vi "STEP LOAD SEQUENCE.vi"(8 "error in (no error)":errorcluster, 11 "main ref":T1) -> (0 "error out":errorcluster)   [LabVIEW 2025]
uses:
  controls/LAB-IQ UI Data.ctl
  STEP LOAD SEQUENCE ENUM.ctl
  HEAVE vi's/Heave Write enum.ctl
  cef93557-1e48-4b46-994d-460df1ebe7ff.vi
panel:
  out "ELAPSED TIMER":dbl
  out "Test Size":i32
  in  "Time Index":i32
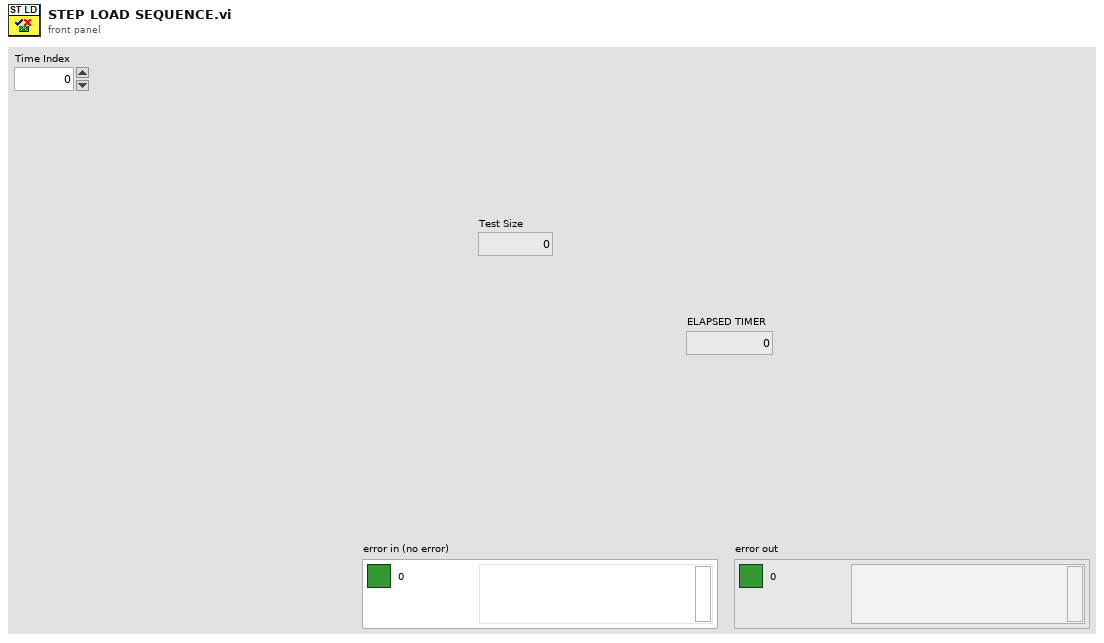
[diagram p1: front panel]
types:
  T1 = typedef "LAB-IQ UI Data.ctl" = cluster{"Main Home Screen":cluster{"GUI":refnum<vi>, "Platform Settings":refnum<vi>, "Configure":refnum<vi>, "Home":refnum<vi>, "EXIT":refnum<vi>, "service 2":refnum<vi>, "MainPage":refnum<vi>, "Analysis":refnum<vi>}, "Platform Settings":cluster{"mm/s  Surge":refnum<vi>, "Update Surge Speed":refnum<vi>, "Drive Error":refnum<vi>, "Disable Axis Jog Soft Limits":refnum<vi>, "mm/s  Sway":refnum<vi>, "Sway and Surge COM Status":refnum<vi>, "Heave COM Status":refnum<vi>, "Enable Platform":refnum<vi>, "Surge Forward Main":refnum<vi>, "Sway Right Main":refnum<vi>, "Sway Left Main":refnum<vi>, "Heave Down Main":refnum<vi>, "Heave Up main":refnum<vi>, "Update Sway Speed":refnum<vi>, "Update Heave Speed":refnum<vi>, "mm/s Heave":refnum<vi>, "mm/sec":refnum<vi>, "mm":refnum<vi>, "Surge Backward Main":refnum<vi>}, "Analysis Screen":cluster{"Analysis Home":refnum<vi>, "Surface Analysis":refnum<vi>, "Imaging":refnum<vi>, "Image Analysis":refnum<vi>, "Post Analysis":refnum<vi>}, "Config Screen":cluster{"Select Load Head":refnum<vi>, "Notes :":refnum<vi>, "FILE":refnum<vi>, "Sample ID :":refnum<vi>, "Operator ID :":refnum<vi>, "Operator Name :":refnum<vi>, "Auto":refnum<vi>}, "Motion Module":cluster{"zNL":refnum<vi>, "NL disp":refnum<vi>, "Rotary Tab":refnum<vi>, "Motion Direction:  3":refnum<vi>, "E.Velocity 2":refnum<vi>, "e.v/ssr 2":refnum<vi>, "Enter Fixed E.Velocity 2":refnum<vi>, "Enter Final SRR 2":refnum<vi>, "Enter initial SRR 2":refnum<vi>, "Enter Fixed SRR 2":refnum<vi>, "Enter the Final E.Velocity (m/s) 2":refnum<vi>, "Enter initial E.Velocity (m/s) 2":refnum<vi>, "Final Speed (RPM) 3":refnum<vi>, "Initial Speed (RPM) 2":refnum<vi>, "Enter the Final Velocity (m/s) 3":refnum<vi>, "Enter initial Velocity (m/s)  3":refnum<vi>, "Ramp Up 2":refnum<vi>, "TEST SELECTION":refnum<vi>, "SPEED SELECTION : ":refnum<vi>, "Angular Oscillation Set":refnum<vi>, "Traction":refnum<vi>, "Step Speed":refnum<vi>, "StepTable For Load-Speed":refnum<vi>, "StepTable For Speed":refnum<vi>, "Surge Forward MM":refnum<vi>, "Surge Backward MM":refnum<vi>, "M3 Image":refnum<vi>, "String 39":refnum<vi>, "Sway Left MM":refnum<vi>, "Sway Right MM":refnum<vi>, "Disable Axis Jog Soft Limits":refnum<vi>, "mm":refnum<vi>, "Heave Down MM":refnum<vi>, "Heave Up MM":refnum<vi>, "Wear Track Diameter (mm)":refnum<vi>, "Set WTD":refnum<vi>, "HomeScratch":refnum<vi>, "HomeRot":refnum<vi>, "PlaceModule":refnum<vi>, "Enter the Angle (Deg)":refnum<vi>, "Enter the Frequency (Hz)":refnum<vi>, "Motion Mode:":refnum<vi>, "LR Sway":refnum<vi>, "Rot Hor":refnum<vi>, "Scratch":refnum<vi>, "LR Cam":refnum<vi>, "MMBack":refnum<vi>, "MMNext":refnum<vi>, "Rot Ver":refnum<vi>, "Rotary Module Selection":refnum<vi>, "calculate rotary":refnum<vi>, "SPEED SELECTION : rotary":refnum<vi>, "Import 2":refnum<vi>, "Save 2":refnum<vi>, "File Path :  2":refnum<vi>, "String 45":refnum<vi>, "StepTable For Speed 3":refnum<vi>, "Enter the Speed(mm/sec)":refnum<vi>, "Enter the Speed(RPM)":refnum<vi>, "Enter Scratch Speed (mm/s):":refnum<vi>, "SwaySpeed Set":refnum<vi>, "Scartch Offset":refnum<vi>, "Motion type:":refnum<vi>, "HomeScratch 2":refnum<vi>, "Enter Scratch length (mm):":refnum<vi>, "Wear Track Diameter":refnum<vi>, "Rotary Speed Exced":refnum<vi>, "Scratch Mode":refnum<vi>, "No of Scratch":refnum<vi>}, "Environmental control":cluster{"Humidity  Status  3":refnum<vi>, "Low Temp  Status  2":refnum<vi>, "TK4 status 2":refnum<vi>, "Stage Temperature":refnum<vi>, "Sample Temperature":refnum<vi>, "Humidity (Amb)":refnum<vi>, "Clear List":refnum<vi>, "Add to list":refnum<vi>, "Wear":refnum<vi>, "Vibration":refnum<vi>, "Humidity (Chamber)":refnum<vi>, "Temperature (Chamber)":refnum<vi>, "ECR ":refnum<vi>, "Temperature (Amb)":refnum<vi>, "Microphone":refnum<vi>, "Acoustic Emission 3":refnum<vi>, "SNext":refnum<vi>, "APBack":refnum<vi>, "Enter the Temperature (°C):":refnum<vi>, "Enter the Stage \nTemperature (°C):":refnum<vi>, "Enter the Humidity (%Rh):":refnum<vi>, "Low Temp":refnum<vi>, "High Temp":refnum<vi>, "Humidity":refnum<vi>, "Sensors Picked":refnum<vi>}, "About Screen":cluster{"Password":refnum<vi>, "Home Service":refnum<vi>, "Advanced Setting":refnum<vi>, "About Tab":refnum<vi>, "ECR Port:":refnum<vi>, "Ramp Port:":refnum<vi>, "Installation/Replacement completed":refnum<vi>, "Loahead":refnum<vi>, "Heave and Surge COM Port:":refnum<vi>, "Sway COM Port:":refnum<vi>, "Temp Modbus:":refnum<vi>, "Humidity Port:":refnum<vi>, "Edit Gain Constants":refnum<vi>, "Save Gain Constants":refnum<vi>}, "Main Screen":cluster{"Main Screen Tab":refnum<vi>, "Angle and Frequency":refnum<vi>, "Stroke (mm)":refnum<vi>, "Angle (Deg)":refnum<vi>, "Main Speed Tab":refnum<vi>, "MTM MOTOR DISPLAY":refnum<vi>, "Disc Speed (m/sec)":refnum<vi>, "Ball Speed (m/sec)":refnum<vi>, "Disc Speed (RPM)":refnum<vi>, "Ball Speed (RPM)":refnum<vi>, "SPEED TAB":refnum<vi>, "Speed (m/sec)":refnum<vi>, "Set Speed (m/sec)":refnum<vi>, "Speed (RPM)":refnum<vi>, "Set Speed":refnum<vi>, "Time Tab":refnum<vi>, "Time ( HH:MM:SS ) 2":refnum<vi>, "Test Duration":refnum<vi>, "Test Duration 4":refnum<vi>, "TEST CYCLE":refnum<vi>, "TOTAL CYCLES":refnum<vi>, "Set Load (N)":refnum<vi>, "Temp Tabs":refnum<vi>, "Heater":refnum<vi>, "TK4 status":refnum<vi>, "ChamberTemp":refnum<vi>, "SetTmp":refnum<vi>, "Controller  Status":refnum<vi>, "ChamberTemp 2":refnum<vi>, "SetTmp 2":refnum<vi>, "Controller  Status 2":refnum<vi>, "ChamberTemp 3":refnum<vi>, "SetTmp 3":refnum<vi>, "Cooling":refnum<vi>, "Load Communication":refnum<vi>, "Ambient \nTemperature":refnum<vi>, "HumCOMStatus":refnum<vi>, "Ambient\n Humidity":refnum<vi>, "Freq (Hz)":refnum<vi>, "Load En":refnum<vi>, "NLt":refnum<vi>, "zNL 2":refnum<vi>, "Humidity On":refnum<vi>, "humidity disp":refnum<vi>, "Set Humidity":refnum<vi>, "NL disp 2":refnum<vi>, "Humidity On 2":refnum<vi>, "humidity disp 2":refnum<vi>, "Set Humidity 2":refnum<vi>, "NL disp 3":refnum<vi>, "AppLoadSeq scratch":refnum<vi>, "Stop Scratch":refnum<vi>, "ClrLog":refnum<vi>, "Trip Log":refnum<vi>, "STOP":refnum<vi>, "Start Test":refnum<vi>, "Test status":refnum<vi>, "AR Led":refnum<vi>, "Data":refnum<vi>, "Health":refnum<vi>, "Sway COM Status":refnum<vi>, "Heave COM Status":refnum<vi>, "Grp Tab":refnum<vi>, "Sub Graph":refnum<vi>, "SD (mm)":refnum<vi>, "Siliding distance Reset Graph":refnum<vi>, "SDGp":refnum<vi>, "Humidity Reset Graph":refnum<vi>, "HumrGp":refnum<vi>, "Acoustic Emission (mV)":refnum<vi>, "Aqucostic Reset Graph":refnum<vi>, "gACQUOS":refnum<vi>, "ECR RESET":refnum<vi>, "ECR":refnum<vi>, "Temperature Reset":refnum<vi>, "Acoustic Emission (mV) 2":refnum<vi>, "Aqucostic Reset Graph 2":refnum<vi>, "gACQUOS 2":refnum<vi>, "ECR RESET 2":refnum<vi>, "ECR 2":refnum<vi>, "Temperature Reset 2":refnum<vi>, "Temperature (deg c)":refnum<vi>, "Speed Reset Graph":refnum<vi>, "Speed Tab":refnum<vi>, "MTM DISC  SPEED":refnum<vi>, "MTM BALL SPEED":refnum<vi>, "speed mm/sec":refnum<vi>, "Hymidity":refnum<vi>, "Humidity Disable trip":refnum<vi>, "CoF Trip  2":refnum<vi>, "Depth Trip":refnum<vi>, "Weart Deapth":refnum<vi>, "Depth Reset Graph":refnum<vi>, "Weart":refnum<vi>, "Depthz":refnum<vi>, "Depth (µm)":refnum<vi>, "WearGp":refnum<vi>, "NL Trip 2":refnum<vi>, "Load pid":refnum<vi>, "Load Disable Trip":refnum<vi>, "Load Reset Graph":refnum<vi>, "NL Display 4":refnum<vi>, "Main Chart 3":refnum<vi>, "BACK":refnum<vi>, "Depth Trip 2":refnum<vi>, "COF TRIP ":refnum<vi>, "Friction Force (N)":refnum<vi>, "FF Reset Graph":refnum<vi>, "FF Disable Trip":refnum<vi>, "FF TRIP":refnum<vi>, "COF Disable Trip":refnum<vi>, "COF Reset Graph":refnum<vi>, "Start Test Temp":refnum<vi>, "zFF":refnum<vi>, "Friction Force (N) Graph":refnum<vi>, "Coefficient of Friction":refnum<vi>, "Scratch Start Test":refnum<vi>, "FF Tab":refnum<vi>, "Cyclic Friction Force (N)":refnum<vi>, "CZ FF":refnum<vi>, "Cyclic Friction Force (N) Graph":refnum<vi>, "Cyclic Coefficient of Friction":refnum<vi>, "Cyclic FF TRIP":refnum<vi>, "Cyclic FF Disable Trip":refnum<vi>, "cyclic COF Disable Trip":refnum<vi>, "cyclic COF TRIP":refnum<vi>, "cyclic COF Reset Graph":refnum<vi>, "Cyclic FF Reset Graph":refnum<vi>, "Test Trip":refnum<vi>, "Multi Scratch Pass":refnum<vi>}, "Loading":cluster{"Indentation":refnum<vi>, "Reference Sample":refnum<vi>, "Load Cell Communication Slide":refnum<vi>, "com 3":refnum<vi>, "com":refnum<vi>, "DecaForce COM Status":refnum<vi>, "Update":refnum<vi>, "Clear 3":refnum<vi>, "seq":refnum<vi>, "Stribeck table":refnum<vi>, "Stribeck Table  For loading":refnum<vi>, "Loading Mode":refnum<vi>, "Enter the Final Load (N)":refnum<vi>, "Enter the CoF Trip":refnum<vi>, "Enter the Friction Force Trip":refnum<vi>, "Enter the Normal load Trip":refnum<vi>, "Enter the Load  (N)":refnum<vi>, "KiloForce":refnum<vi>, "DecaForce ":refnum<vi>, "MicroForce":refnum<vi>, "LHBack":refnum<vi>, "LHNext":refnum<vi>, "Enter the Loading Rate (N/min)":refnum<vi>, "Message":refnum<vi>, "Warning 2":refnum<vi>, "SSP 0.75":refnum<vi>, "SSP 0.5":refnum<vi>, "SSP 0.3":refnum<vi>, "Warning":refnum<vi>, "gui GIF":refnum<vi>, "Communication is established":refnum<vi>, "AppLoad 4":refnum<vi>, "Multipoint":refnum<vi>, "Load Selection":refnum<vi>}, "PID":cluster{"Ramp MulFac":refnum<vi>, "pulses LoadDiffRamp(2..10)":refnum<vi>, "PulseControlRamp(diff<=3N)":refnum<vi>, "SetLoadDeadband(%) Load(0-10N)":refnum<vi>, "PID gains out delay (microForce)":refnum<vi>, "Ramp":refnum<vi>, "Gain 2":refnum<vi>, "pulses LoadDiff(2..10)":refnum<vi>, "pulses LoadDiff(11..50)":refnum<vi>, "PulseControl(diff<=3N)":refnum<vi>, "SetLoadDeadband(%)  2":refnum<vi>, "Dummy Run":refnum<vi>, "Vertical load (N)":refnum<vi>, "AutoTune":refnum<vi>, "Offset 3 ":refnum<vi>, "apply load":refnum<vi>, "Offset  3":refnum<vi>, "apply load 2":refnum<vi>, "Enter ByPass Load":refnum<vi>, "reinit 3":refnum<vi>, "output range delay":refnum<vi>, "PID gains out delay":refnum<vi>, "Bypass Load":refnum<vi>, "pulsesSent":refnum<vi>, "pulses ":refnum<vi>, "actpid":refnum<vi>, "gFF Rot":refnum<vi>, "pulses LoadDiff(21..1000)":refnum<vi>, "Delay":refnum<vi>, "deadband":refnum<vi>}, "Config Parameters":cluster{"Tab Control 3":refnum<vi>, "Tab Control 19":refnum<vi>, "SAMPLES":refnum<vi>, "Re-initilaize":refnum<vi>, "Filter ON/OFF":refnum<vi>, "TracHomeSurgeOffsetCounts 10MM":refnum<vi>, "TracHomeSwayOffsetCounts 10MM":refnum<vi>, "Acoustic Emission:":refnum<vi>, "Apply Filter (FF)":refnum<vi>, "Filter% 2":refnum<vi>, "Apply Filter (Load)":refnum<vi>, "Filter% ":refnum<vi>, "Sway distance (mm)":refnum<vi>, "Surge distance (mm)":refnum<vi>, "DataSavingLoopDelay(ms)":refnum<vi>, "SAVE 2":refnum<vi>, "Enter Distance":refnum<vi>, "Sway Counts:":refnum<vi>, "Distance (mm): 3":refnum<vi>, "Surge Counts:":refnum<vi>, "Distance (mm): 2":refnum<vi>, "Distance (mm):":refnum<vi>, "Heave Counts:":refnum<vi>, "LRMHomeSurgeOffsetCounts":refnum<vi>, "LRMHomeSwayOffsetCounts":refnum<vi>, "TracHomeSurgeOffsetCounts 20MM":refnum<vi>, "TracHomeSwayOffsetCounts 20MM":refnum<vi>, "RotHomeSwayOffsetCounts":refnum<vi>, "RotHomeSurgeOffsetCounts":refnum<vi>, "Heave distance":refnum<vi>, "Zmm":refnum<vi>, "Heave Pulses/mm":refnum<vi>, "Surge Pulses/mm":refnum<vi>, "Sway Pulses/mm":refnum<vi>, "Heave Pitch":refnum<vi>, "Surge Pitch":refnum<vi>, "Sway Pitch":refnum<vi>, "Heave PPR":refnum<vi>, "Surge PPR":refnum<vi>, "Sway PPR":refnum<vi>, "Tab Control 5":refnum<vi>, "Tab Control 14":refnum<vi>, "Tab Control 26":refnum<vi>, "AE":refnum<vi>, "Heave Loop Delay":refnum<vi>, "Heave PID Speed":refnum<vi>, "Surge Jog Speed":refnum<vi>, "Heave Jog Speed":refnum<vi>, "Sway Loop Delay":refnum<vi>, "Sway PID Speed":refnum<vi>, "Sway Jog Speed":refnum<vi>}, "Loading Com Port":cluster{"ClearAll":refnum<vi>, "Mz(Nm)":refnum<vi>, "My(Nm)":refnum<vi>, "Mx(Nm)":refnum<vi>, "Save Dwell":refnum<vi>, "Mx ":refnum<vi>, "My ":refnum<vi>, "Mz":refnum<vi>, "Fx(N)":refnum<vi>, "Fy(N)":refnum<vi>, "Fz(N)":refnum<vi>, "ZeroAll":refnum<vi>, "Acq Delay (ms)":refnum<vi>, "Burst Delay (ms)":refnum<vi>, "model":refnum<vi>, "SN":refnum<vi>, "FFx(N)":refnum<vi>, "Sensor IP":refnum<vi>, "Port":refnum<vi>, "FFy(N)":refnum<vi>, "Load(N)":refnum<vi>, "delete Handle":refnum<vi>, "Create Handle":refnum<vi>, "ft_data":refnum<vi>, "ft_range":refnum<vi>, "ft_data 2":refnum<vi>, "stop 6":refnum<vi>, "running_flag":refnum<vi>, "ft_udp_handle":refnum<vi>, "get-data-return":refnum<vi>, "get-range-return":refnum<vi>, "zero-return":refnum<vi>, "filter-return":refnum<vi>, "initial-return":refnum<vi>, "deleteHandle-result":refnum<vi>, "Load Cell Temp":refnum<vi>}, "Heave AND Surge":cluster{"SURGE POSE":refnum<vi>, "error out Read":refnum<vi>, "HEAVE POSE":refnum<vi>, "State":refnum<vi>, "Homed":refnum<vi>, "Sequence ID":refnum<vi>, "error out Write":refnum<vi>, "faultCode":refnum<vi>, "Ack ID":refnum<vi>, "SPEED":refnum<vi>, "Distance":refnum<vi>, "Mode Command":refnum<vi>, "Heave and Surge Read":refnum<vi>, "Read Heave Temp":refnum<vi>, "Spare 15":refnum<vi>, "Spare 14":refnum<vi>, "Spare 13":refnum<vi>, "Spare 12":refnum<vi>, "Spare 11":refnum<vi>, "Spare 10":refnum<vi>, "Spare 9":refnum<vi>, "Spare 8":refnum<vi>, "Spare 7":refnum<vi>, "Spare 6":refnum<vi>, "Spare 5":refnum<vi>, "Spare 4":refnum<vi>, "Spare 2":refnum<vi>, "Spare 1":refnum<vi>, "Node Id":refnum<vi>, "Spare 3":refnum<vi>, "SPARE 4":refnum<vi>, "SPARE 3":refnum<vi>, "SPARE 2":refnum<vi>, "SPARE 1":refnum<vi>, "fwMajor":refnum<vi>, "fwMinor":refnum<vi>, "Manual Write":refnum<vi>, "Heave and Surge Write":refnum<vi>}, "New PID LOGIC":cluster{"Fine Tune Zone":refnum<vi>, "PID SDelay":refnum<vi>, "Max_pos_limit":refnum<vi>, "Min_pos_limit":refnum<vi>, "i_limit":refnum<vi>, "pct_scale":refnum<vi>, "Deadband":refnum<vi>, "Kd":refnum<vi>, "Ki":refnum<vi>, "Kp":refnum<vi>, "Current Position":refnum<vi>, "Set Load":refnum<vi>, "Current Load":refnum<vi>, "Pulse delta":refnum<vi>, "Init Step":refnum<vi>, "Max Step Linit":refnum<vi>}, "SWAY ":cluster{"fwMajor":refnum<vi>, "Homed":refnum<vi>, "Rotary POSE":refnum<vi>, "State":refnum<vi>, "SWAY POSE":refnum<vi>, "Ack ID":refnum<vi>, "faultCode":refnum<vi>, "Node Id":refnum<vi>, "fwMinor":refnum<vi>, "Spare 6":refnum<vi>, "Spare 5":refnum<vi>, "Spare 4":refnum<vi>, "Spare 3":refnum<vi>, "Spare 2":refnum<vi>, "Spare 1":refnum<vi>, "Spare 7":refnum<vi>, "SPARE  5":refnum<vi>, "error out Write  SWAY ":refnum<vi>, "error out Read SWAY ":refnum<vi>, "Manual Write SWAY ":refnum<vi>, "SWAY WRITE":refnum<vi>, "SPARE  4":refnum<vi>, "SPARE  3":refnum<vi>, "SPARE 2":refnum<vi>, "SPARE 1":refnum<vi>, "Spare 15":refnum<vi>, "Spare 14":refnum<vi>, "Spare 13":refnum<vi>, "Spare 12":refnum<vi>, "Spare 11":refnum<vi>, "Spare 9":refnum<vi>, "Spare 8":refnum<vi>, "SPEED":refnum<vi>, "Distance":refnum<vi>, "Mode Command":refnum<vi>, "Sequence ID":refnum<vi>, "SWAY READ":refnum<vi>, "Spare 10":refnum<vi>, "Read SWAY Temp":refnum<vi>}, "Analysis Screen":cluster{"Analysis Home":refnum<vi>, "Refresh 2":refnum<vi>, "MEAN 4":refnum<vi>, "SD 4":refnum<vi>, "VARIANCE 4":refnum<vi>, "MEAN  3":refnum<vi>, "SD  3":refnum<vi>, "VARIANCE  3":refnum<vi>, "MEAN 2":refnum<vi>, "SD  2":refnum<vi>, "VARIANCE 2":refnum<vi>, "MEAN":refnum<vi>, "SD":refnum<vi>, "VARIANCE":refnum<vi>, "File 4 Discription":refnum<vi>, "OPEN 4":refnum<vi>, "File Name 4":refnum<vi>, "OPEN 3":refnum<vi>, "File 3 Discription":refnum<vi>, "File Name 3":refnum<vi>, "Y-AXIS":refnum<vi>, "X-AXIS":refnum<vi>, "XY Graph":refnum<vi>, "File Name 2":refnum<vi>, "File Name 1":refnum<vi>, "OPEN 2":refnum<vi>, "OPEN 1":refnum<vi>, "File 1 Discription ":refnum<vi>, "File 2 Discription":refnum<vi>}}
  T2 = enum32{"Setup", "Load Head", "Motion Module", "Environment", "Begin"}
  T3 = typedef "STEP LOAD SEQUENCE ENUM.ctl" = enum16{"INIT", "TEST START", "TEST INCREMENT", "TEST STOP"}
  T4 = typedef "Heave Write enum.ctl" = enum16{"INIT", "WRITE", "CLOSE", "REINIT"}
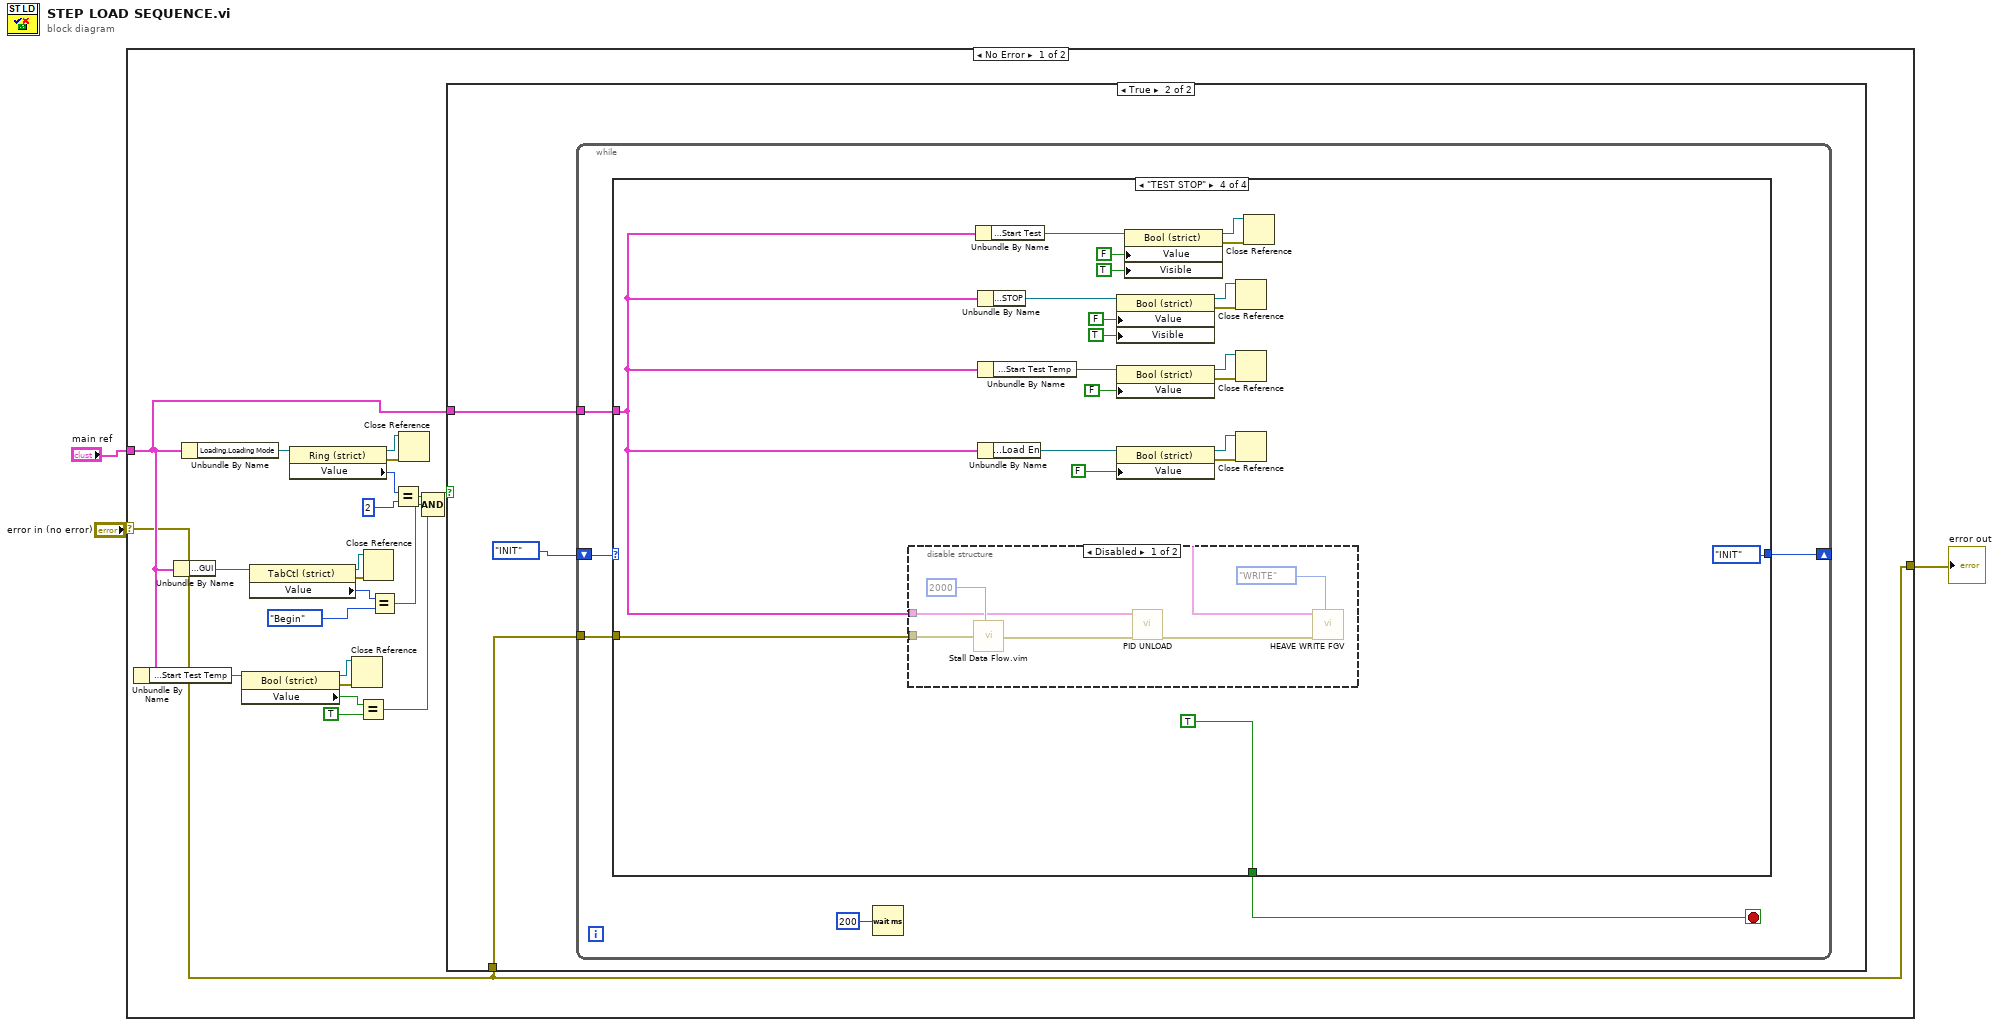
[diagram p0: block diagram]
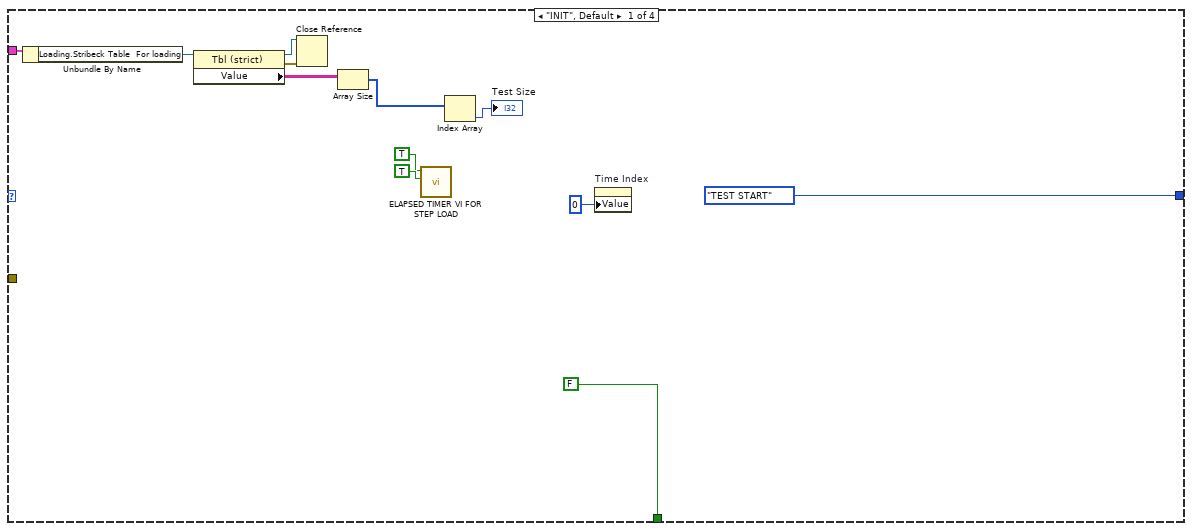
[diagram p3: hidden frame]
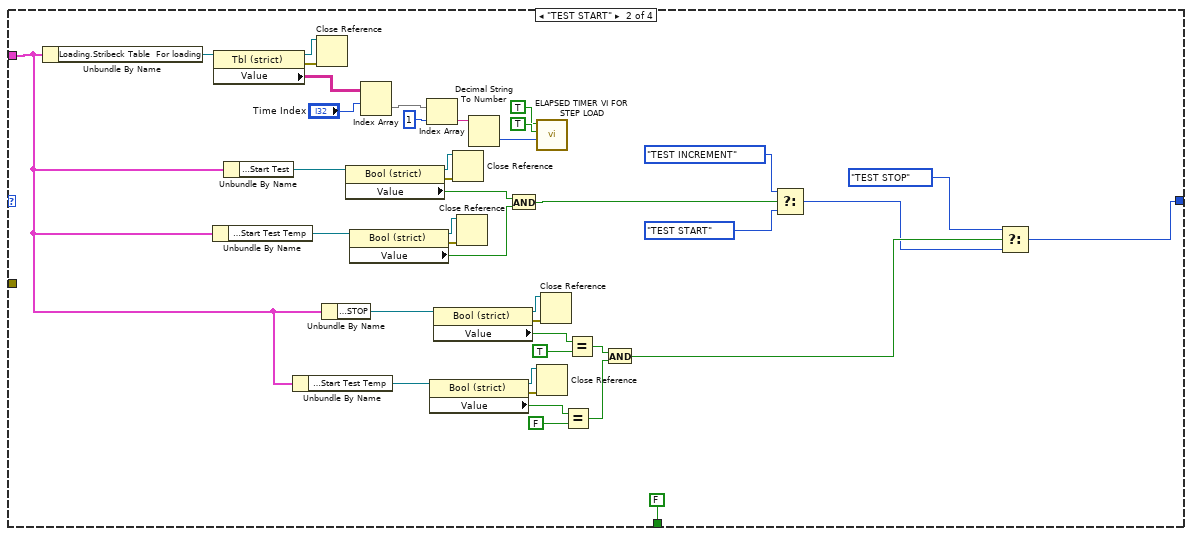
[diagram p4: hidden frame]
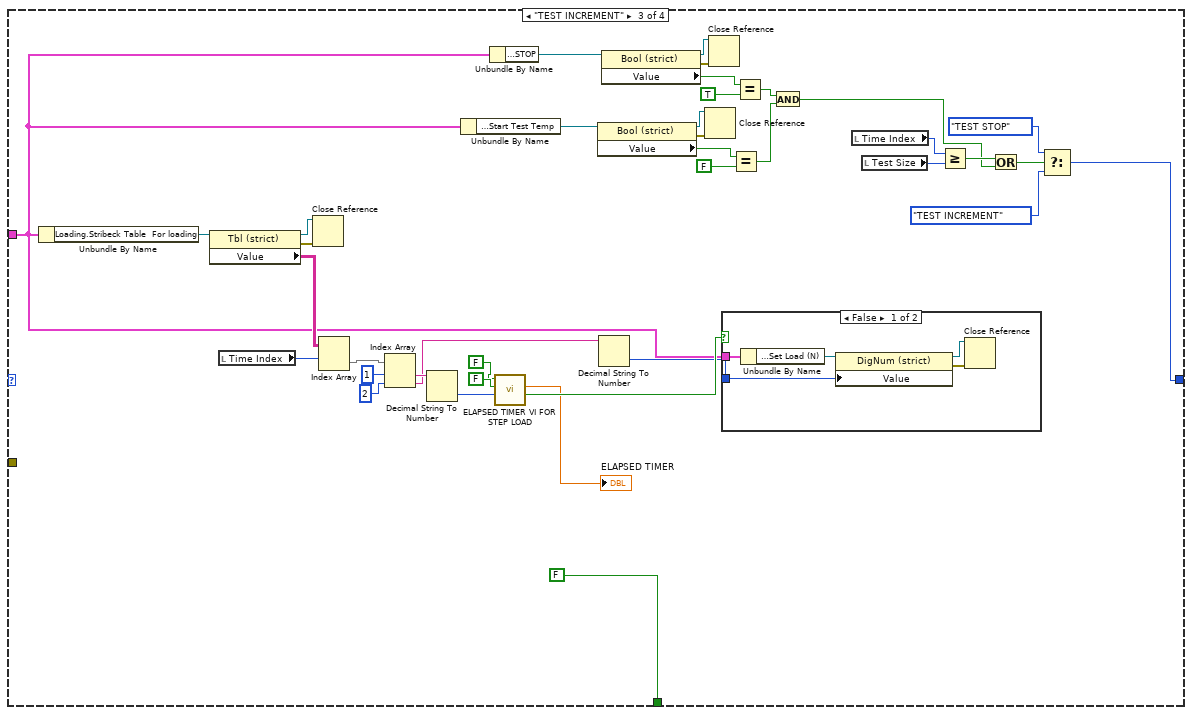
[diagram p5: hidden frame]
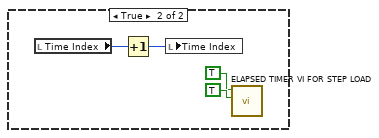
[diagram p6: hidden frame]
diagram:
  n1 = case shown="No Error" "error in (no error)" {
    selector: "error in (no error)" -> [w4 _]
    tunnel: "main ref" -> [w7 _]
    tunnel: [w4 _] -> w1
    frame No Error {
      n2 = Unbundle By Name(w7) -> ("Main Screen.Start Test Temp"=w10:refnum<vi>)
      n3 = Unbundle By Name(w7) -> ("Main Home Screen.GUI"=w16:refnum<vi>)
      n4 = Unbundle By Name(w7) -> ("Loading.Loading Mode"=w24:refnum<vi>)
      n5 = property class="Bool (strict)"(reference=w10) -> (reference out=w8:refnum<vi>, error out=w9:errorcluster, "Value"=w11:bool)  [unwired: 1 in]
      n6 = property class="TabCtl (strict)"(reference=w16) -> (reference out=w18:refnum<vi>, error out=w17:errorcluster, "Value"=w14:T2)  [unwired: 1 in]
      n7 = property class="Ring (strict)"(reference=w24) -> (reference out=w22:refnum<vi>, error out=w23:errorcluster, "Value"=w21:u16)  [unwired: 1 in]
      n8 = Close Reference(reference=w8, error in (no error)=w9) -> ()  [unwired: 1 out]
      n9 = Equal?(x=w11, y=TRUE) -> (x = y?=w6:bool)
      n10 = Close Reference(reference=w18, error in (no error)=w17) -> ()  [unwired: 1 out]
      n11 = Equal?(x=w14, y=T2."Begin" ("Value")) -> (x = y?=w12:bool)
      n12 = Equal?(x=w21, y=u16 2 ("Value")) -> (x = y?=w19:bool)
      n13 = Close Reference(reference=w22, error in (no error)=w23) -> ()  [unwired: 1 out]
      n14 = Compound Arithmetic op=AND(w19, w12, w6) -> (w15:bool)
      n15 = case shown="True" w15 {
        tunnel: w7 -> [_ w26]
        tunnel: w4 -> [_ w25]
        frame False {
        }
        frame True {
          n16 = while {
            shift-right: [w32] -> _
            shift-left: STEP_LOAD_SEQUENCE_ENUM."INIT" -> [w33]
            tunnel: w26 -> [w30]
            tunnel: w25 -> [w29]
            stop <- w31 stop-if-true
            n17 = case shown="\"TEST STOP\"" w33 {
              tunnel: [STEP_LOAD_SEQUENCE_ENUM."TEST START" w46 w106 STEP_LOAD_SEQUENCE_ENUM."INIT"] -> w32
              tunnel: [FALSE FALSE FALSE TRUE] -> w31
              tunnel: w30 -> [w35 w53 w86 w135]
              tunnel: w29 -> [_ _ _ w140]
              frame "INIT", Default {
                n18 = Unbundle By Name(w35) -> ("Loading.Stribeck Table  For loading"=w38:refnum<vi>)
                n19 = property class="Tbl (strict)"(reference=w38) -> (reference out=w36:refnum<vi>, error out=w37:errorcluster, "Value"=w34:string[][])  [unwired: 1 in]
                n20 = Close Reference(reference=w36, error in (no error)=w37) -> ()  [unwired: 1 out]
                n21 = Array Size(array=w34) -> (size(s)=w41:i32[])
                n22 = call "ELAPSED TIMER VI FOR STEP LOAD.vi"("RESET"=TRUE, "PAUSE"=TRUE) -> ()  [unwired: 7 in, 3 out]
                n23 = Index Array(array=w41) -> (element=→"Test Size":i32)  [unwired: 1 in]
                n24 = property on="Time Index" class="DigNum (strict)"("Value"=0 ("Time Index")) -> ()  [unwired: 2 in, 2 out]
              }
              frame "TEST START" {
                n25 = Unbundle By Name(w53) -> ("Loading.Stribeck Table  For loading"=w76:refnum<vi>)
                n26 = Unbundle By Name(w53) -> ("Main Screen.Start Test Temp"=w69:refnum<vi>)
                n27 = property class="Tbl (strict)"(reference=w76) -> (reference out=w74:refnum<vi>, error out=w75:errorcluster, "Value"=w73:string[][])  [unwired: 1 in]
                n28 = Unbundle By Name(w53) -> ("Main Screen.Start Test"=w70:refnum<vi>)
                n29 = Unbundle By Name(w53) -> ("Main Screen.Start Test Temp"=w56:refnum<vi>)
                n30 = Close Reference(reference=w74, error in (no error)=w75) -> ()  [unwired: 1 out]
                n31 = Unbundle By Name(w53) -> ("Main Screen.STOP"=w61:refnum<vi>)
                n32 = property class="Bool (strict)"(reference=w70) -> (reference out=w72:refnum<vi>, error out=w71:errorcluster, "Value"=w66:bool)  [unwired: 1 in]
                n33 = property class="Bool (strict)"(reference=w69) -> (reference out=w67:refnum<vi>, error out=w68:errorcluster, "Value"=w65:bool)  [unwired: 1 in]
                n34 = Index Array(array=w73, index (row)="Time Index") -> (element=w82:string[])  [unwired: 1 in]
                n35 = Index Array(array=w82, index=1) -> (element=w80:string)
                n36 = property class="Bool (strict)"(reference=w56) -> (reference out=w54:refnum<vi>, error out=w55:errorcluster, "Value"=w57:bool)  [unwired: 1 in]
                n37 = property class="Bool (strict)"(reference=w61) -> (reference out=w63:refnum<vi>, error out=w62:errorcluster, "Value"=w60:bool)  [unwired: 1 in]
                n38 = Close Reference(reference=w72, error in (no error)=w71) -> ()  [unwired: 1 out]
                n39 = Close Reference(reference=w67, error in (no error)=w68) -> ()  [unwired: 1 out]
                n40 = Decimal String To Number(string=w80) -> (number=w77:i32)  [unwired: 2 in, 1 out]
                n41 = And(x=w66, y=w65) -> (x .and. y?=w64:bool)
                n42 = call "ELAPSED TIMER VI FOR STEP LOAD.vi"("TARGET"=w77, "RESET"=TRUE, "PAUSE"=TRUE) -> ()  [unwired: 6 in, 3 out]
                n43 = Close Reference(reference=w54, error in (no error)=w55) -> ()  [unwired: 1 out]
                n44 = Close Reference(reference=w63, error in (no error)=w62) -> ()  [unwired: 1 out]
                n45 = Equal?(x=w57, y=FALSE) -> (x = y?=w51:bool)
                n46 = Equal?(x=w60, y=TRUE) -> (x = y?=w52:bool)
                n47 = And(x=w52, y=w51) -> (x .and. y?=w49:bool)
                n48 = Select(t=STEP_LOAD_SEQUENCE_ENUM."TEST INCREMENT", s=w64, f=STEP_LOAD_SEQUENCE_ENUM."TEST START") -> (s? t:f=w48:T3)
                n49 = Select(t=STEP_LOAD_SEQUENCE_ENUM."TEST STOP", s=w49, f=w48) -> (s? t:f=w46:T3)
              }
              frame "TEST INCREMENT" {
                n50 = Unbundle By Name(w86) -> ("Loading.Stribeck Table  For loading"=w103:refnum<vi>)
                n51 = property class="Tbl (strict)"(reference=w103) -> (reference out=w101:refnum<vi>, error out=w102:errorcluster, "Value"=w100:string[][])  [unwired: 1 in]
                n52 = local read "Time Index"() -> (w123:i32)
                n53 = Close Reference(reference=w101, error in (no error)=w102) -> ()  [unwired: 1 out]
                n54 = Index Array(array=w100, index (row)=w123) -> (element=w118:string[])  [unwired: 1 in]
                n55 = Index Array(array=w118, index #1=1 ("index"), index #2=2 ("index")) -> (element #1=w117:string, element #2=w114:string)
                n56 = Decimal String To Number(string=w117) -> (number=w122:i32)  [unwired: 2 in, 1 out]
                n57 = Unbundle By Name(w86) -> ("Main Screen.Start Test Temp"=w92:refnum<vi>)
                n58 = Unbundle By Name(w86) -> ("Main Screen.STOP"=w97:refnum<vi>)
                n59 = call "ELAPSED TIMER VI FOR STEP LOAD.vi"("TARGET"=w122, "RESET"=FALSE, "PAUSE"=FALSE) -> ("ELAPSED INDICATION"=w116:bool, "ELAPSED TIMER"=→"ELAPSED TIMER":dbl)  [unwired: 6 in, 1 out]
                n60 = property class="Bool (strict)"(reference=w92) -> (reference out=w90:refnum<vi>, error out=w91:errorcluster, "Value"=w93:bool)  [unwired: 1 in]
                n61 = Decimal String To Number(string=w114) -> (number=w105:i32)  [unwired: 2 in, 1 out]
                n62 = property class="Bool (strict)"(reference=w97) -> (reference out=w99:refnum<vi>, error out=w98:errorcluster, "Value"=w96:bool)  [unwired: 1 in]
                n63 = Close Reference(reference=w90, error in (no error)=w91) -> ()  [unwired: 1 out]
                n64 = Close Reference(reference=w99, error in (no error)=w98) -> ()  [unwired: 1 out]
                n65 = case shown="False" w116 {
                  tunnel: w105 -> [w124 _]
                  tunnel: w86 -> [w125 _]
                  frame False {
                    n66 = Unbundle By Name(w125) -> ("Main Screen.Set Load (N)"=w128:refnum<vi>)
                    n67 = property class="DigNum (strict)"(reference=w128, "Value"=w124) -> (reference out=w126:refnum<vi>, error out=w127:errorcluster)  [unwired: 1 in]
                    n68 = Close Reference(reference=w126, error in (no error)=w127) -> ()  [unwired: 1 out]
                  }
                  frame True {
                    n69 = local read "Time Index"() -> (w132:i32)
                    n70 = Increment(x=w132) -> (x+1=w131:i32)
                    n71 = local write "Time Index"(w131) -> ()
                    n72 = call "ELAPSED TIMER VI FOR STEP LOAD.vi"("RESET"=TRUE, "PAUSE"=TRUE) -> ()  [unwired: 7 in, 3 out]
                  }
                }
                n73 = Equal?(x=w93, y=FALSE) -> (x = y?=w88:bool)
                n74 = Equal?(x=w96, y=TRUE) -> (x = y?=w89:bool)
                n75 = And(x=w89, y=w88) -> (x .and. y?=w87:bool)
                n76 = local read "Time Index"() -> (w112:i32)
                n77 = local read "Test Size"() -> (w111:i32)
                n78 = Greater Or Equal?(x=w112, y=w111) -> (x >= y?=w110:bool)
                n79 = Or(x=w110, y=w87) -> (x .or. y?=w109:bool)
                n80 = Select(t=STEP_LOAD_SEQUENCE_ENUM."TEST STOP", s=w109, f=STEP_LOAD_SEQUENCE_ENUM."TEST INCREMENT") -> (s? t:f=w106:T3)
              }
              frame "TEST STOP" {
                n81 = disable-structure shown="Disabled" {
                  disable-tunnel: w140 -> [w156 _]
                  disable-tunnel: w135 -> [w155 _]
                  frame Disabled {
                    n82 = call "Stall Data Flow.vim"("value in"=w156, "milliseconds to wait"=u32 2000) -> ("value out"=w158:errorcluster)  [unwired: 1 out]
                    n83 = call "PID UNLOAD.vi"("error in (no error)"=w158, "main ref"=w155) -> ("error out"=w159:errorcluster)  [unwired: 9 in]
                    n84 = call "HEAVE WRITE FGV.vi"("Enum - Menu"=Heave_Write_enum."WRITE", "error in (no error)"=w159, "main ref"=w155) -> ()  [unwired: 8 in, 1 out]
                  }
                  frame Enabled {
                  }
                }
                n85 = Unbundle By Name(w135) -> ("Main Screen.Start Test"=w138:refnum<vi>)
                n86 = Unbundle By Name(w135) -> ("Main Screen.STOP"=w150:refnum<vi>)
                n87 = Unbundle By Name(w135) -> ("Main Screen.Start Test Temp"=w149:refnum<vi>)
                n88 = Unbundle By Name(w135) -> ("Main Screen.Load En"=w141:refnum<vi>)
                n89 = property class="Bool (strict)"(reference=w150, "Value"=FALSE, "Visible"=TRUE) -> (reference out=w152:refnum<vi>, error out=w151:errorcluster)  [unwired: 1 in]
                n90 = property class="Bool (strict)"(reference=w149, "Value"=FALSE) -> (reference out=w147:refnum<vi>, error out=w148:errorcluster)  [unwired: 1 in]
                n91 = property class="Bool (strict)"(reference=w141, "Value"=FALSE) -> (reference out=w143:refnum<vi>, error out=w142:errorcluster)  [unwired: 1 in]
                n92 = property class="Bool (strict)"(reference=w138, "Value"=FALSE, "Visible"=TRUE) -> (reference out=w136:refnum<vi>, error out=w137:errorcluster)  [unwired: 1 in]
                n93 = Close Reference(reference=w152, error in (no error)=w151) -> ()  [unwired: 1 out]
                n94 = Close Reference(reference=w147, error in (no error)=w148) -> ()  [unwired: 1 out]
                n95 = Close Reference(reference=w143, error in (no error)=w142) -> ()  [unwired: 1 out]
                n96 = Close Reference(reference=w136, error in (no error)=w137) -> ()  [unwired: 1 out]
              }
            }
            n97 = Wait (ms)(milliseconds to wait=u32 200) -> ()  [unwired: 1 out]
          }
        }
      }
    }
    frame Error {
    }
  }
  "error out" <- w1
